vi "02rutas_archivos.vi"(5 "DAT PATH":path) -> (0 "CANT EQ":i64, 1 "ALARMAS":i64[](array[numeric]), 2 "sound":bool, 3 "ULTIMA FECHA":dbl[](array[numeric]), 4 "block":bool, 6 "DATA PATH":string, 8 "ESTADOS":i64[](array[numeric]), 9 "NOMBRES":string[](array[string]), 10 "error out":errorcluster)   [LabVIEW 2010]
uses:
  <vilib>/Utility/file.llb/Read From Spreadsheet File (I64).vi
  <vilib>/Utility/file.llb/Read From Spreadsheet File (string).vi
  <vilib>/Utility/file.llb/Read From Spreadsheet File (DBL).vi
panel:
  out "refnum out":refnum<file>
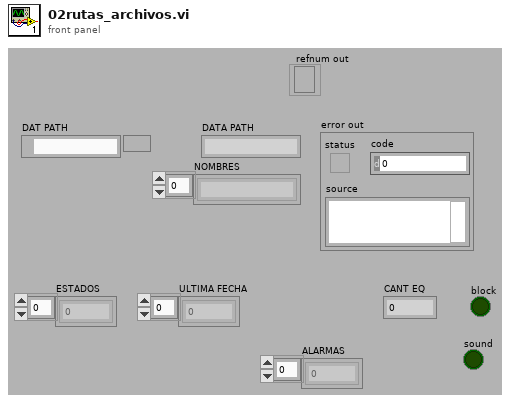
[diagram p1: front panel]
types:
  T1 = enum16{"open", "replace", "create", "open or create", "replace or create", "replace or create with confirmation"}
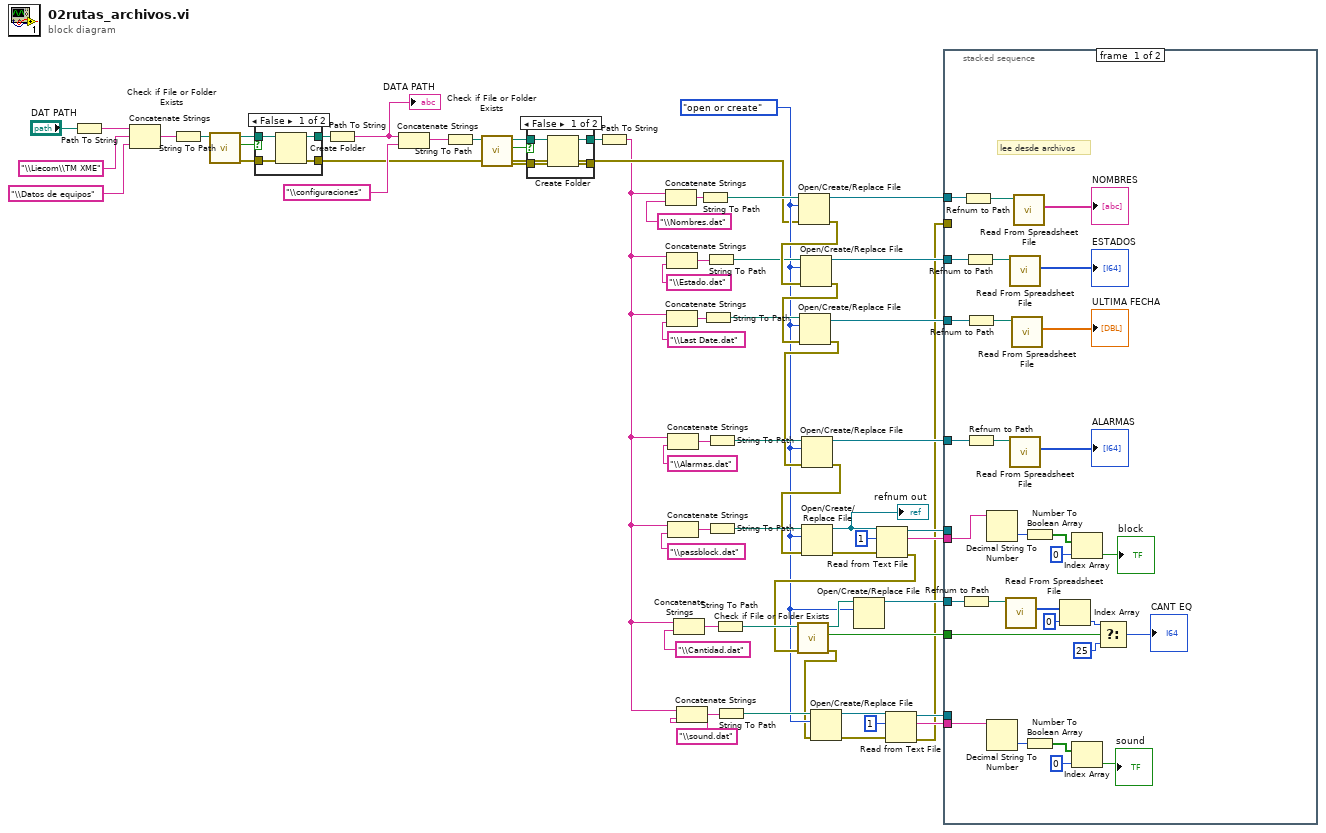
[diagram p0: block diagram]
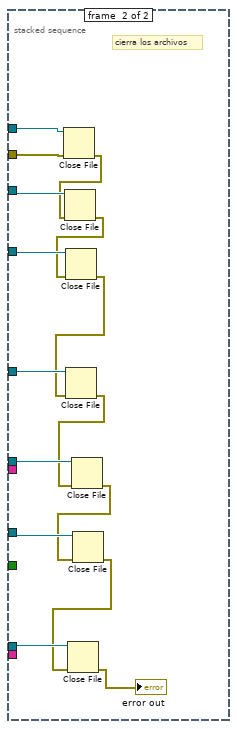
[diagram p3: hidden frame]
diagram:
  w14 = T1."open or create" ("operation (0:open)")
  n1 = Path To String(path="DAT PATH") -> (string=w11:string)
  n2 = Concatenate Strings(w11, "\\Liecom\\TM XME" ("search string"), "\\Datos de equipos" ("search string")) -> (w66:string)
  n3 = String To Path(string=w66) -> (path=w59:path)
  n4 = call <vilib>:"Check if File or Folder Exists.vi"("path"=w59) -> ("error out"=w65:errorcluster, "file or folder exists?"=w60:bool, "dup path"=w61:path)  [unwired: 1 in, 7 out]
  n5 = case shown="False" w60 {
    tunnel: w61 -> [w70 w72]
    tunnel: [w69 w72] -> w62
    tunnel: w65 -> [w68 w71]
    tunnel: [w67 w71] -> w12
    frame False {
      n6 = Create Folder(path (use dialog)=w70, error in=w68) -> (created path=w69:path, error out=w67:errorcluster)  [unwired: 2 out]
    }
    frame True {
    }
  }
  n7 = Path To String(path=w62) -> (string=w29:string)
  "DATA PATH" <- w29
  n8 = Concatenate Strings(w29, "\\configuraciones") -> (w3:string)
  n9 = String To Path(string=w3) -> (path=w8:path)
  n10 = call <vilib>:"Check if File or Folder Exists.vi"("path"=w8) -> ("error out"=w4:errorcluster, "file or folder exists?"=w7:bool, "dup path"=w6:path)  [unwired: 1 in, 7 out]
  n11 = case shown="False" w7 {
    tunnel: w6 -> [w76 w78]
    tunnel: [w75 w78] -> w5
    tunnel: w4 -> [w74 w77]
    tunnel: [w73 w77] -> _
    frame False {
      n12 = Create Folder(path (use dialog)=w76, error in=w74) -> (created path=w75:path, error out=w73:errorcluster)  [unwired: 2 out]
    }
    frame True {
    }
  }
  n13 = Path To String(path=w5) -> (string=w2:string)
  n14 = Concatenate Strings(w2, "\\Nombres.dat") -> (w47:string)
  n15 = Concatenate Strings(w2, "\\Estado.dat") -> (w46:string)
  n16 = Concatenate Strings(w2, "\\Last Date.dat") -> (w45:string)
  n17 = Concatenate Strings(w2, "\\Alarmas.dat") -> (w26:string)
  n18 = Concatenate Strings(w2, "\\passblock.dat") -> (w39:string)
  n19 = Concatenate Strings(w2, "\\Cantidad.dat") -> (w52:string)
  n20 = Concatenate Strings(w2, "\\sound.dat") -> (w18:string)
  n21 = String To Path(string=w47) -> (path=w41:path)
  n22 = String To Path(string=w45) -> (path=w44:path)
  n23 = String To Path(string=w46) -> (path=w43:path)
  n24 = String To Path(string=w26) -> (path=w25:path)
  n25 = String To Path(string=w39) -> (path=w38:path)
  n26 = String To Path(string=w52) -> (path=w56:path)
  n27 = String To Path(string=w18) -> (path=w19:path)
  n28 = Open/Create/Replace File(file path (use dialog)=w41, error in=w12, operation (0:open)=w14) -> (refnum out=w40:refnum<file>, error out=w63:errorcluster)  [unwired: 4 out]
  n29 = Open/Create/Replace File(file path (use dialog)=w43, error in=w63, operation (0:open)=w14) -> (refnum out=w50:refnum<file>, error out=w64:errorcluster)  [unwired: 4 out]
  n30 = Open/Create/Replace File(file path (use dialog)=w44, error in=w64, operation (0:open)=w14) -> (refnum out=w51:refnum<file>, error out=w23:errorcluster)  [unwired: 4 out]
  n31 = Open/Create/Replace File(file path (use dialog)=w25, error in=w23, operation (0:open)=w14) -> (refnum out=w28:refnum<file>, error out=w24:errorcluster)  [unwired: 4 out]
  n32 = Open/Create/Replace File(file path (use dialog)=w38, error in=w24, operation (0:open)=w14) -> (refnum out=w36:refnum<file>, error out=w33:errorcluster)  [unwired: 4 out]
  "refnum out" <- w36
  n33 = Read from Text File(file (use dialog)=w36, count=1, error in=w33) -> (refnum out=w34:refnum<file>, text=w35:string, error out=w32:errorcluster)  [unwired: 1 in, 1 out]
  n34 = call <vilib>:"Check if File or Folder Exists.vi"("error in (no error)"=w32, "path"=w56) -> ("error out"=w13:errorcluster, "file or folder exists?"=w57:bool, "dup path"=w58:path)  [unwired: 7 out]
  n35 = Open/Create/Replace File(file path (use dialog)=w19, error in=w13, operation (0:open)=w14) -> (refnum out=w20:refnum<file>, error out=w21:errorcluster)  [unwired: 4 out]
  n36 = Open/Create/Replace File(file path (use dialog)=w58, operation (0:open)=w14) -> (refnum out=w54:refnum<file>)  [unwired: 1 in, 5 out]
  n37 = Read from Text File(file (use dialog)=w20, count=1, error in=w21) -> (refnum out=w16:refnum<file>, text=w17:string, error out=w1:errorcluster)  [unwired: 1 in, 1 out]
  n38 = stacked-sequence {
    tunnel: w57 -> [w102 _]
    tunnel: w54 -> [w98 w123]
    tunnel: w51 -> [w97 w122]
    tunnel: w50 -> [w96 w121]
    tunnel: w40 -> [w93 w120]
    tunnel: w35 -> [w87 _]
    tunnel: w34 -> [_ w119]
    tunnel: w28 -> [w86 w118]
    tunnel: w17 -> [w79 _]
    tunnel: w16 -> [_ w117]
    tunnel: w1 -> [_ w109]
    frame #0 {
      # "lee desde archivos"
      n39 = Refnum to Path(1:w98) -> (0:w99:path)
      n40 = Refnum to Path(1:w93) -> (0:w92:path)
      n41 = Refnum to Path(1:w96) -> (0:w94:path)
      n42 = Refnum to Path(1:w97) -> (0:w95:path)
      n43 = Refnum to Path(1:w86) -> (0:w85:path)
      n44 = Decimal String To Number(string=w87) -> (number=w91:i32)  [unwired: 2 in, 1 out]
      n45 = Decimal String To Number(string=w79) -> (number=w80:i32)  [unwired: 2 in, 1 out]
      n46 = call-poly <vilib>:"Read From Spreadsheet File.vi"("file path (dialog if empty)"=w99) -> ("first row"=w100:i64[])  [unwired: 3 in, 7 out]
      n47 = call-poly <vilib>:"Read From Spreadsheet File.vi"("file path (dialog if empty)"=w94) -> ("first row"=→"ESTADOS":i64[])  [unwired: 3 in, 7 out]
      n48 = call-poly <vilib>:"Read From Spreadsheet File.vi"("file path (dialog if empty)"=w85) -> ("first row"=→"ALARMAS":i64[])  [unwired: 3 in, 7 out]
      n49 = call-poly <vilib>:"Read From Spreadsheet File.vi"("file path (dialog if empty)"=w95) -> ("first row"=→"ULTIMA FECHA":dbl[])  [unwired: 3 in, 7 out]
      n50 = call-poly <vilib>:"Read From Spreadsheet File.vi"("file path (dialog if empty)"=w92) -> ("first row"=→"NOMBRES":string[])  [unwired: 3 in, 7 out]
      n51 = Number To Boolean Array(number=w91) -> (Boolean array=w90:bool[])
      n52 = Number To Boolean Array(number=w80) -> (Boolean array=w81:bool[])
      n53 = Index Array(array=w100, index=0) -> (element=w103:i64)
      n54 = Index Array(array=w90, index=0) -> (element=→"block":bool)
      n55 = Index Array(array=w81, index=0) -> (element=→"sound":bool)
      n56 = Select(t=w103, s=w102, f=i64 25) -> (s? t:f=→"CANT EQ":i64)
    }
    frame #1 {
      # "cierra los archivos"
      n57 = Close File(refnum=w120, error in=w109) -> (error out=w116:errorcluster)  [unwired: 1 out]
      n58 = Close File(refnum=w121, error in=w116) -> (error out=w115:errorcluster)  [unwired: 1 out]
      n59 = Close File(refnum=w122, error in=w115) -> (error out=w114:errorcluster)  [unwired: 1 out]
      n60 = Close File(refnum=w118, error in=w114) -> (error out=w113:errorcluster)  [unwired: 1 out]
      n61 = Close File(refnum=w119, error in=w113) -> (error out=w112:errorcluster)  [unwired: 1 out]
      n62 = Close File(refnum=w123, error in=w112) -> (error out=w111:errorcluster)  [unwired: 1 out]
      n63 = Close File(refnum=w117, error in=w111) -> (error out=→"error out":errorcluster)  [unwired: 1 out]
    }
  }
